vi "Set Full SPI Engine Configuration 256-bit.vi"(7 "Chip Select":u8, 8 "error in":errorcluster, 9 "Set? (T)":bool=TRUE, 10 "SPI Physical Settings":T1={"Divide Value"=0, "Transfer Length (bits)"=1, "CS Asserted Polarity"=FALSE, "Clock Polarity (CPOL)"=FALSE, "Clock Phase (CPHA)"=FALSE, "Lengthen MISO Setup"=FALSE, "Direction Change Bit"=0, "MOSI Starts as Output"=FALSE, "Tristatable MOSI"=FALSE} {"Direction Change Bit" max=64 step=1; "Transfer Length (bits)" min=1 max=64 step=1}, 11 "SPI Engine Resources":T2={"To SPI Engine Data FIFO"="DLU To SPI Engine Data FIFO", "From SPI Engine Data FIFO"="SPI Engine to DLU Data FIFO", "Data to SPI Engine Cache Register"="Data to SPI Engine (Cache)", "SPI Transaction Settings Cache Register"="SPI PHY Settings to SPI Engine (Cache)"}) -> (0 "error out":errorcluster, 3 "SPI Engine Resources":T2={"To SPI Engine Data FIFO"="DLU To SPI Engine Data FIFO", "From SPI Engine Data FIFO"="SPI Engine to DLU Data FIFO", "Data to SPI Engine Cache Register"="Data to SPI Engine (Cache)", "SPI Transaction Settings Cache Register"="SPI PHY Settings to SPI Engine (Cache)"})   [LabVIEW 2015, in "SPI API.lvlib"]
doc: "This VI Configures SPI Settings for the required channel (using Chip Select ID) on SPI bus."
uses:
  SPI API.lvlib
  Controls/SPI Engine Resources 256-bit.ctl
  Custom SPI IP/Controls/Custom SPI IP U16 Transfer Settings.ctl
  Controls/SPI Transaction Settings U16.ctl
  <vilib>/rvi/DataTransferAndStorage/Container/Common/niFpgaContainerExecOnDevCompGetState.vi
  <vilib>/rvi/Emulation/niFpgaEmulationIsFPGAContextNoSignature.vi
  <vilib>/rvi/DataTransferAndStorage/Container/Common/niFpgaContainerGetUniqueNameForEmu.vi
  <vilib>/rvi/Memory/Memory_Emulation/niFpgaMemoryEmulationCacheClearOnFirstRun.vi
  <vilib>/rvi/Memory/Memory_Emulation/nirvimemoryEmulationManagerCache_MakeExclusive.vi
  <vilib>/rvi/Memory/Memory_Emulation/niFpgaMemoryEmulationValidateCache.vi
  <vilib>/rvi/Memory/Memory_Emulation/nirvimemoryEmulationManagerCache_InsertValue.vi
  <vilib>/Utility/error.llb/Clear Errors.vi
  <vilib>/rvi/Memory/Memory_Emulation/nirvimemoryEmulationManagerCache_ReleaseExclusive.vi
  <vilib>/rvi/Memory/Memory_Emulation/nirvimemoryEmulationManagerCache_GetValue.vi
  <vilib>/rvi/Memory/Memory_Emulation/nirvimemoryEmulationManagerCache_SetValue.vi
  <vilib>/rvi/Emulation/niFpgaProcessEmulError.vi
  <vilib>/rvi/Emulation/niFpgaSctlEmulationGetInTimedLoop.vi
  <vilib>/rvi/DataTransferAndStorage/Container/XNode/niFpgaContainer.xnode
  <vilib>/rvi/DataTransferAndStorage/Register/Emulation/niFpgaRegisterEmulationRefIn.vi
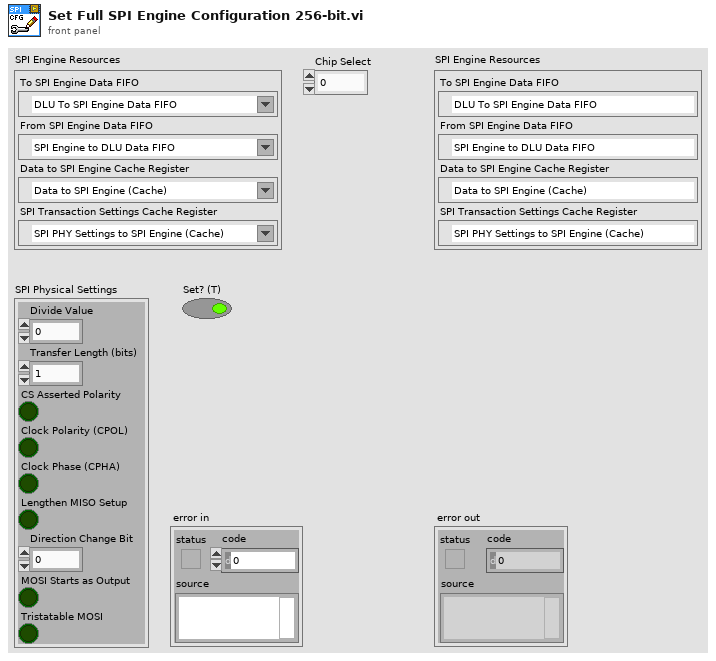
[diagram p1: front panel]
types:
  T1 = typedef "SPI API.lvlib/Custom SPI IP U16 Transfer Settings.ctl" = cluster{"Divide Value":u8, "Transfer Length (bits)":u16, "CS Asserted Polarity":bool, "Clock Polarity (CPOL)":bool, "Clock Phase (CPHA)":bool, "Lengthen MISO Setup":bool, "Direction Change Bit":u8, "MOSI Starts as Output":bool, "Tristatable MOSI":bool}
  T2 = typedef "SPI API.lvlib/SPI Engine Resources 256-bit.ctl" = cluster{"To SPI Engine Data FIFO":refnum<k21>, "From SPI Engine Data FIFO":refnum<k21>, "Data to SPI Engine Cache Register":refnum<k21>, "SPI Transaction Settings Cache Register":refnum<k21>}
  T3 = typedef "SPI API.lvlib/SPI Transaction Settings U16.ctl" = cluster{"Chip Select ID":u8, "SPI Physical Settings":T1}
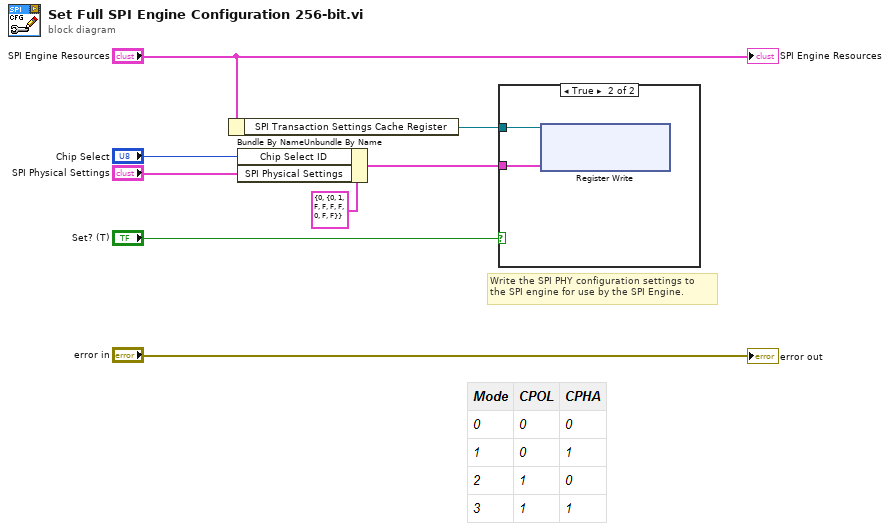
[diagram p0: block diagram]
diagram:
  # "Write the SPI PHY configuration settings to\nthe SPI engine for use by the SPI Engine."
  n1 = Unbundle By Name("SPI Engine Resources") -> ("SPI Transaction Settings Cache Register"=w6:refnum<k21>)
  n2 = Bundle By Name(cluster=T3 {"Chip Select ID"=0, "SPI Physical Settings"={"Divide Value"=0, "Transfer Length (bits)"=1, "CS Asserted Polarity"=FALSE, "Clock Polarity (CPOL)"=FALSE, "Clock Phase (CPHA)"=FALSE, "Lengthen MISO Setup"=FALSE, "Direction Change Bit"=0, "MOSI Starts as Output"=FALSE, "Tristatable MOSI"=FALSE}} ("SPI Settings"), "Chip Select ID"="Chip Select", "SPI Physical Settings"="SPI Physical Settings") -> (w5:T3)
  n3 = case shown="True" "Set? (T)" {
    tunnel: w6 -> [_ w10]
    tunnel: w5 -> [_ w9]
    frame False {
    }
    frame True {
      n4 = xnode "Register Write"("Data"=w9, "Register In"=w10) -> ()  [unwired: 1 out]
    }
  }
  "error out" <- "error in"
  "SPI Engine Resources" <- "SPI Engine Resources"
